vi "Wavelet Packet - Split Node.vi"() -> ()   [LabVIEW 2023]
doc: "This example shows how to split a terminal node of a wavelet packet tree with the WA WP Split VI.\n\n<b>Instructions:</b>\nRun this VI. Define a terminal node to split."
uses:
  <vilib>/addons/Wavelet Analysis/typedefs.llb/WA Data.ctl
  <vilib>/addons/Wavelet Analysis/wavelet packet.llb/WA WP Decomposition (Waveform).vi
  <vilib>/addons/_Advanced Signal Processing/NI_AdvSigProcWA.lvlib
panel:
  in  "stop":bool
  out "Wavelet Packet Tree":picture
  in  "Node to split":string="001"
  # "Overview: Shows how to split a terminal node of a wavelet packet tree with the WA WP Split VI.\nRequirements: LabVIEW Full Development System, Advanced Signal Processing Toolkit\nInstructions: \n1. Run this VI. Define a terminal node to split.\n2. Click Stop to stop the VI."
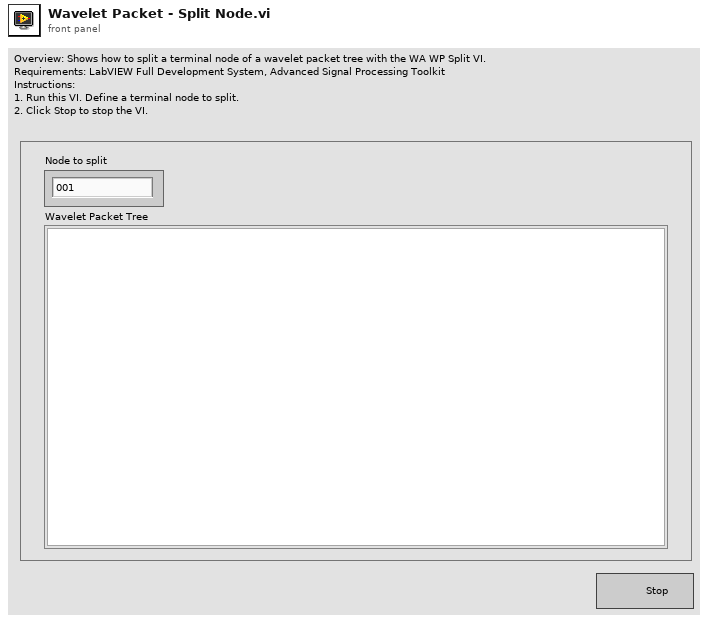
[diagram p1: front panel]
types:
  T1 = typedef "NI_AdvSigProcWA.lvlib/WA Data.ctl" = u16
  T2 = typedef "NI_AdvSigProcWA.lvlib/WA Generic Ref.ctl" = cluster{"ref":u64, "t0":timestamp, "dt":dbl}
  T3 = typedef "LVBoundsTypeDef.ctl" = cluster{"Width":u32, "Height":u32}
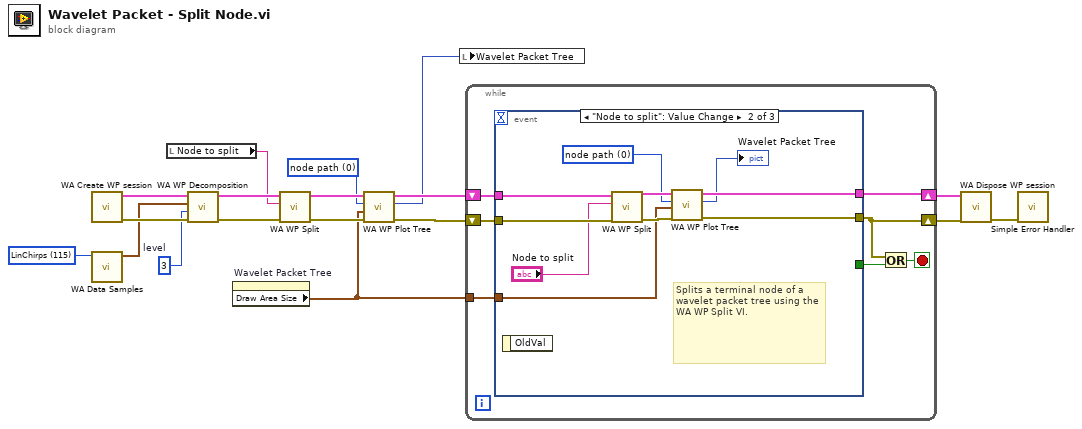
[diagram p0: block diagram]
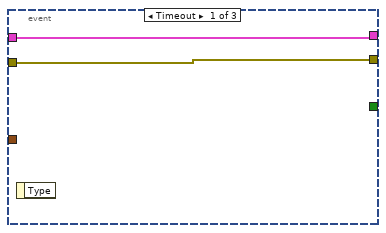
[diagram p2: hidden frame]
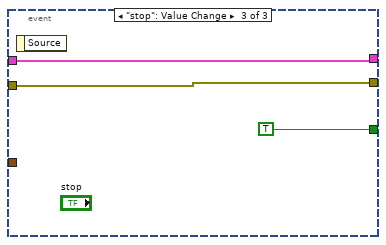
[diagram p3: hidden frame]
diagram:
  w4 = T1 115 items=["1D Example Data"=100, "-"=101, "Doppler"=102, "HOP"=103, "TF Sine"=104, "Noisy Doppler"=105, "Sea Temperature"=106, "Sp500"=107, "Power Line"=108, "Engine Knocking"=109, "HeaviSine"=110, "Bumps"=111, "Blocks"=112, "Piece Regular"=113, "HypChirps"=114, "LinChirps"=115, "Chirps"=116, "Piece Polynomial"=117, "ECG"=131, "-"=118, "2D Example Data"=119, "-"=120, "Finger Print (Image)"=121, "Iris Flower (Image)"=122, "Mammogram (Image)"=123, "Lake (Image)"=127, "Two Can 1 (Image)"=132, "Two Can 2 (Image)"=133, "Camera Man (Image)"=134] ("data")
  w7 = u16 0 items=["node path", "(depth, pos)", "entropy"] ("display mode")
  w11 = 3  # level
  n1 = call <vilib>:"WA Create WP session.vi"() -> ("error out"=w17:errorcluster, "WP session out"=w18:T2)  [unwired: 1 in, 9 out]
  n2 = call <vilib>:"WA Data Samples.vi"("data"=w4) -> ("signal"=w12:waveform(dbl))  [unwired: 10 out]
  n3 = local read "Node to split"() -> (w5:string)
  n4 = call-poly <vilib>:"WA WP Decomposition.vi"("error in (no error)"=w17, "levels"=w11, "signal"=w12, "WP session"=w18) -> ("error out"=w15:errorcluster, "WP session out"=w16:T2)  [unwired: 1 in, 5 out]
  n5 = property on="Wavelet Packet Tree" class="Pict"() -> ("Draw Area Size"=w8:T3)  [unwired: 2 in, 2 out]
  n6 = call <vilib>:"WA WP Split.vi"("error in (no error)"=w15, "path"=w5, "WP session"=w16) -> ("error out"=w13:errorcluster, "WP session out"=w14:T2)  [unwired: 1 in, 6 out]
  n7 = call <vilib>:"WA WP Plot Tree.vi"("error in (no error)"=w13, "draw area size"=w8, "display mode"=w7, "WP session"=w14) -> ("error out"=w9:errorcluster, "tree plot"=w6:picture, "WP session out"=w10:T2)  [unwired: 5 out]
  n8 = local write "Wavelet Packet Tree"(w6) -> ()
  n9 = while {
    tunnel: w8 -> [w23]
    shift-right: [w20] -> w2
    shift-left: w10 -> [w25]
    shift-right: [w19] -> w1
    shift-left: w9 -> [w24]
    stop <- w21 stop-if-true
    n10 = event shown="[1] \"Node to split\": Value Change" {
      selector: _ -> [_ _ _]
      dyn-events: _ -> [_ _ _]
      timeout: _ -> [_ _ _]
      tunnel: w25 -> [w27 w36 w39]
      tunnel: w24 -> [w26 w35 w38]
      tunnel: [_ _ TRUE ("error?")] -> w22
      tunnel: [w27 w33 w39] -> w20
      tunnel: w23 -> [_ w31 _]
      tunnel: [w26 w28 w38] -> w19
      event Timeout {
        n11 = event-data() -> ()  [unwired: 2 out]
      }
      event "Node to split": Value Change {
        w29 = u16 0 items=["node path", "(depth, pos)", "entropy"] ("display mode")
        # "Splits a terminal node of a wavelet packet tree using the WA WP Split VI."
        n12 = event-data() -> ()  [unwired: 2 out]
        n13 = call <vilib>:"WA WP Split.vi"("error in (no error)"=w35, "path"="Node to split", "WP session"=w36) -> ("error out"=w34:errorcluster, "WP session out"=w37:T2)  [unwired: 1 in, 6 out]
        n14 = call <vilib>:"WA WP Plot Tree.vi"("error in (no error)"=w34, "draw area size"=w31, "display mode"=w29, "WP session"=w37) -> ("error out"=w28:errorcluster, "tree plot"=→"Wavelet Packet Tree":picture, "WP session out"=w33:T2)  [unwired: 5 out]
      }
      event "stop": Value Change {
        n15 = event-data() -> ()  [unwired: 2 out]
      }
    }
    n16 = Or(x=w19, y=w22) -> (x .or. y?=w21:bool)
  }
  n17 = call <vilib>:"WA Dispose WP session.vi"("error in (no error)"=w1, "WP session"=w2) -> ("error out"=w3:errorcluster)  [unwired: 9 out]
  n18 = call <vilib>:"Simple Error Handler.vi"("error in (no error)"=w3) -> ()  [unwired: 1 in, 8 out]
